vi "Default Instrument Setup.vi"(8 "error in (no error)":errorcluster, 11 "VISA resource name":refnum<visa-resource-name>) -> (0 "error out":errorcluster, 3 "VISA resource name out":refnum<visa-resource-name>)   [LabVIEW 2025]
doc: "Sends a default command string to the instrument whenever a new VISA session is opened, or the instrument is reset. Use this VI as a subVI for the <b>Initialize</b> and <b>Reset</b> VIs. Altering this VI could cause these two VIs to operate incorrectly."
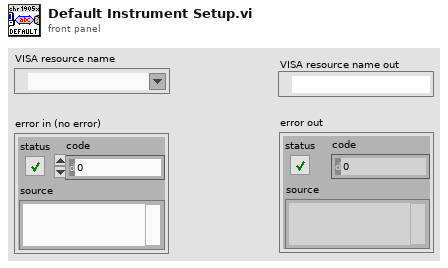
[diagram p1: front panel]
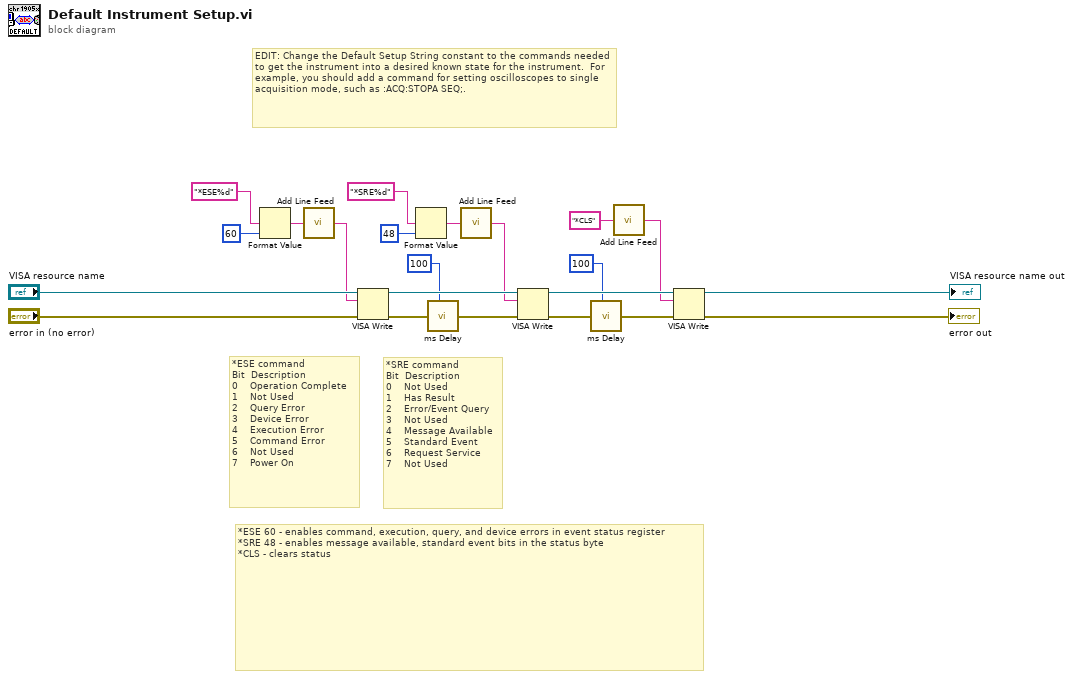
[diagram p0: block diagram]
diagram:
  # "*SRE command\nBit  Description\n0    Not Used\n1    Has Result\n2    Error/Event Query\n3    Not Used\n4    Message Available\n5    Standard Event\n6    Request Service\n7    Not Used"
  # "*ESE command\nBit  Description\n0    Operation Complete\n1    Not Used\n2    Query Error\n3    Device Error\n4    Execution Error\n5    Command Error\n6    Not Used\n7    Power On"
  # "*ESE 60 - enables command, execution, query, and device errors in event status register\n*SRE 48 - enables message available, standard event bits in the status byte\n*CLS - clears status"
  # "EDIT: Change the Default Setup String constant to the commands needed to get the instrument into a desired known state for the instrument.  For example, you should add a command for setting oscilloscopes to single acquisition mode, such as :ACQ:STOPA SEQ;."
  n1 = Format Value(format string="*ESE%d", value (0)=i16 60 ("decimal")) -> (output string=w19:string)  [unwired: 1 in]
  n2 = call "Add Line Feed.vi"("Command string"=w19) -> ("Concatenated string"=w11:string)  [unwired: 4 in]
  n3 = VISA Write(VISA resource name="VISA resource name", write buffer=w11, error in (no error)="error in (no error)") -> (VISA resource name out=w22:refnum<visa-resource-name>, error out=w5:errorcluster)  [unwired: 1 out]
  n4 = Format Value(format string="*SRE%d", value (0)=u32 48 ("value")) -> (output string=w17:string)  [unwired: 1 in]
  n5 = call "ms Delay.vi"("miliseconds to wait"=u32 100 ("milliseconds to wait"), "error in (no error)"=w5) -> ("error out"=w4:errorcluster)  [unwired: 6 in, 1 out]
  n6 = call "Add Line Feed.vi"("Command string"=w17) -> ("Concatenated string"=w14:string)  [unwired: 4 in]
  n7 = VISA Write(VISA resource name=w22, write buffer=w14, error in (no error)=w4) -> (VISA resource name out=w21:refnum<visa-resource-name>, error out=w3:errorcluster)  [unwired: 1 out]
  n8 = call "ms Delay.vi"("miliseconds to wait"=u32 100 ("milliseconds to wait"), "error in (no error)"=w3) -> ("error out"=w2:errorcluster)  [unwired: 6 in, 1 out]
  n9 = call "Add Line Feed.vi"("Command string"="*CLS") -> ("Concatenated string"=w10:string)  [unwired: 4 in]
  n10 = VISA Write(VISA resource name=w21, write buffer=w10, error in (no error)=w2) -> (VISA resource name out=→"VISA resource name out":refnum<visa-resource-name>, error out=→"error out":errorcluster)  [unwired: 1 out]
